vi "BlackBox.vi"(1 "Player Info":T1) -> (0 "Player Info Array":T1[](array[typedef]))   [LabVIEW 2011]
doc: "This Black Box is intended to be used in Homework 2 of the Nigel Says Series. It receives a cluster with the Player Information (Name and Score) and will give back an array of Players Information sorted from Lowest Score to Highest Score."
uses:
  Player Info.ctl
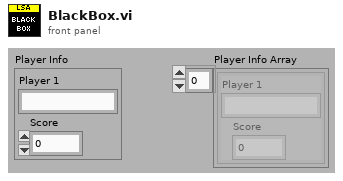
[diagram p1: front panel]
types:
  T1 = typedef "Player Info.ctl" = cluster{"Player 1":string, "Score":i32}
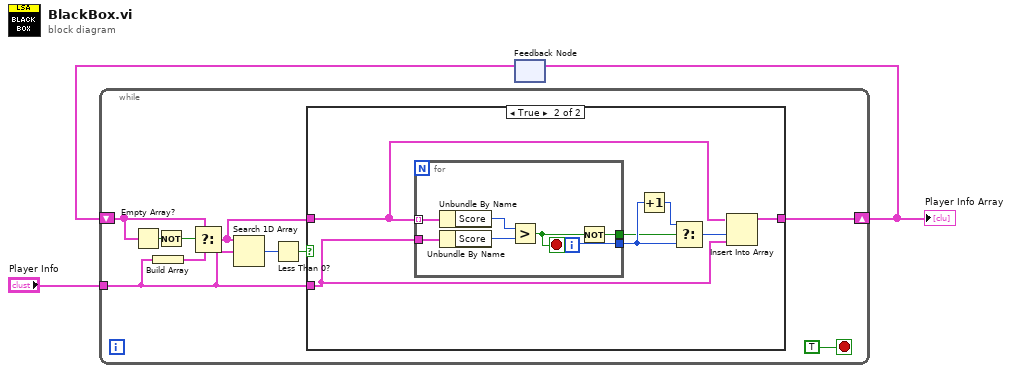
[diagram p0: block diagram]
diagram:
  n1 = feedback #1() -> (w2:T1[])  [unwired: 1 in]
  n2 = while {
    shift-right: [w12] -> w3
    shift-left: w2 -> [w7]
    tunnel: "Player Info" -> [w5]
    stop <- TRUE stop-if-true
    n3 = Empty Array?(array=w7) -> (empty?=w9:bool)
    n4 = Build Array(w5) -> (w6:T1[])
    n5 = Not(x=w9) -> (.not. x?=w8:bool)
    n6 = Select(t=w7, s=w8, f=w6) -> (s? t:f=w4:T1[])
    n7 = Search 1D Array(1D array=w4, element=w5) -> (index of element=w13:i32)  [unwired: 1 in]
    n8 = Less Than 0?(x=w13) -> (x < 0?=w10:bool)
    n9 = case shown="True" w10 {
      tunnel: w4 -> [w14 w20]
      tunnel: w5 -> [_ w19]
      tunnel: [w14 w21] -> w12
      frame False {
      }
      frame True {
        n10 = for {
          tunnel: w20 -> [w24] mode=indexing
          tunnel: w19 -> [w26]
          tunnel: [w28] -> w17
          tunnel: [w23] -> w16
          i -> [w28]
          stop <- w22 stop-if-true
          n11 = Unbundle By Name(w24) -> ("Score"=w25:i32)
          n12 = Unbundle By Name(w26) -> ("Score"=w27:i32)
          n13 = Greater?(x=w25, y=w27) -> (0:w22:bool)
          n14 = Not(x=w22) -> (.not. x?=w23:bool)
        }
        n15 = Increment(x=w17) -> (x+1=w18:i32)
        n16 = Select(t=w18, s=w16, f=w17) -> (s? t:f=w15:i32)
        n17 = Insert Into Array(array=w20, index=w15, new element=w19) -> (w21:T1[])
      }
    }
  }
  "Player Info Array" <- w3
  n18 = feedback-in #1(w3) -> ()
